vi "Fit ASCII Peak.vi"() -> ()   [LabVIEW 2016]
uses:
  <vilib>/Utility/file.llb/Read Delimited Spreadsheet (DBL).vi
  Smooth Background DBL.vi
  <vilib>/Analysis/NI_AALPro.lvlib
panel:
  in  "Use last fit as  guess":bool=TRUE
  in  "Function":enum16{"Gauss", "Lorentz"}(ring)
  out "errors":i32[](array[numeric])
  in  "Signal col":i32=2
  out "Fit":T1(array[cluster])
  in  "Repeat":i32
  in  "Guess":T1(array[cluster])
  in  "Window end":dbl=697.0
  in  "Window start":dbl=690.0
  in  "Filter background":bool=TRUE
  out "Result":T2
  out "error":i32
  out "XY Graph":cluster{"all rows":dbl[], "Data out":dbl[]}[](graph)
  in  "File Path Control":path
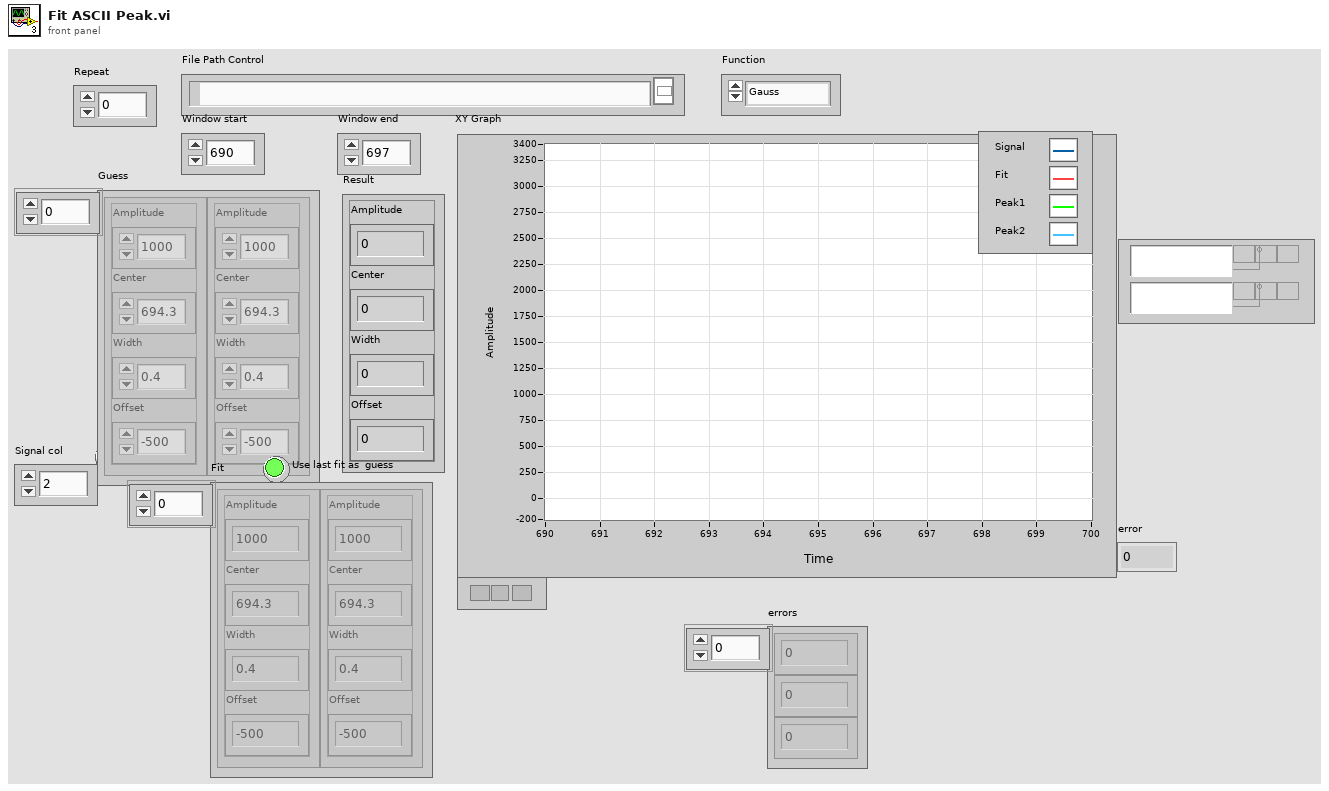
[diagram p1: front panel]
types:
  T1 = cluster{"Amplitude":dbl, "Center":dbl, "Width":dbl, "Offset":dbl}[]
  T2 = cluster{"Amplitude":dbl, "Center":dbl, "Width":dbl, "Offset":dbl}
  T3 = cluster{"amp min":dbl, "amp max":dbl, "center min":dbl, "center max":dbl, "deviation min":dbl, "deviation max":dbl, "offset min":dbl, "offset max":dbl}
  T4 = enum16{"Lowpass", "Highpass", "Bandpass", "Bandstop"}
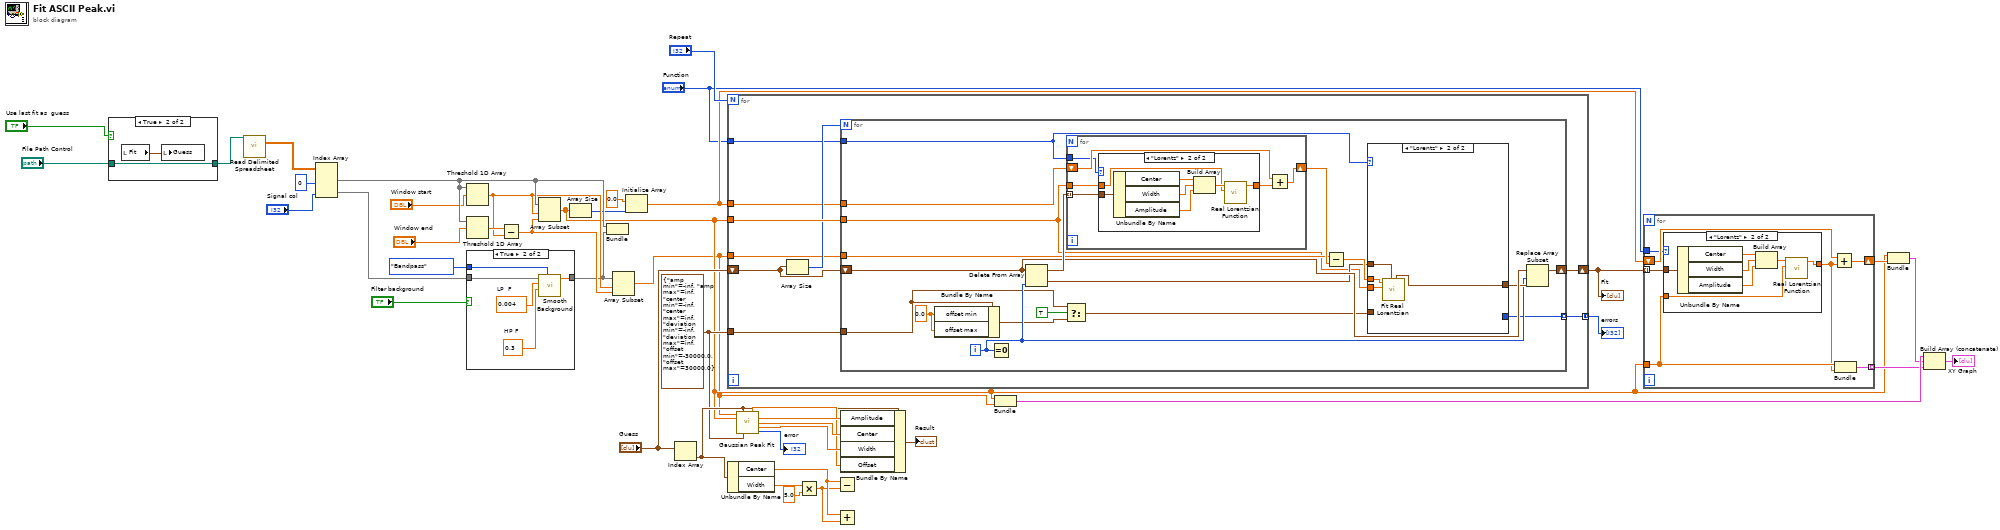
[diagram p0: block diagram]
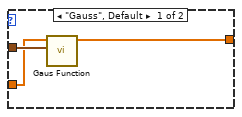
[diagram p3: hidden frame]
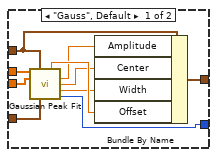
[diagram p4: hidden frame]
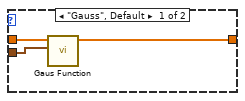
[diagram p5: hidden frame]
diagram:
  w13 = T3 {"amp min"=-inf, "amp max"=inf, "center min"=-inf, "center max"=inf, "deviation min"=-inf, "deviation max"=inf, "offset min"=-30000.0, "offset max"=30000.0} ("parameter bounds")
  n1 = case shown="True" "Use last fit as  guess" {
    tunnel: "File Path Control" -> [w44 w46]
    tunnel: [w44 w46] -> w1
    frame False {
    }
    frame True {
      n2 = local read "Fit"() -> (w45:T1)
      n3 = local write "Guess"(w45) -> ()
    }
  }
  n4 = call-poly <vilib>:"Read Delimited Spreadsheet.vi"("file path (dialog if empty)"=w1) -> ("all rows"=w43:dbl[][])  [unwired: 9 in, 5 out]
  n5 = Index Array(array=w43, index (col) #1=0 ("disabled index (col)"), index (col) #2="Signal col") -> (element #1=w35:dbl[], element #2=w37:dbl[])  [unwired: 2 in]
  n6 = Threshold 1D Array(2:"Window start", 3:w35) -> (0:w33:dbl)  [unwired: 1 in]
  n7 = Threshold 1D Array(2:"Window end", 3:w35) -> (0:w34:dbl)  [unwired: 1 in]
  n8 = case shown="True" "Filter background" {
    tunnel: T4."Bandpass" ("Type") -> [_ w52]
    tunnel: w37 -> [w47 w49]
    tunnel: [w47 w48] -> w31
    frame False {
    }
    frame True {
      w50 = 0.3  # HP F
      w51 = 0.004  # LP  F
      n9 = call-poly "Smooth Background.vi"("Type"=w52, "HP F"=w50, "LP  F"=w51, "Data"=w49) -> ("Data out"=w48:dbl[])  [unwired: 6 in, 1 out]
    }
  }
  n10 = Subtract(x=w34, y=w33) -> (x-y=w32:dbl)
  n11 = Array Subset(array=w35, index=w33, length=w32) -> (w8:dbl[])
  n12 = Array Size(array=w8) -> (size(s)=w16:i32)
  n13 = Bundle("all rows"=w35, "Data out"=w31) -> ()  [unwired: 1 in, 1 out]
  n14 = Array Subset(array=w31, index=w33, length=w32) -> (w6:dbl[])
  n15 = Initialize Array(0.0 ("element"), w16) -> (w10:dbl[])
  n16 = Index Array(array="Guess") -> (element=w18:T2)  [unwired: 1 in]
  n17 = for {
    N: "Repeat" -> [_]
    shift-right: [w56] -> w12
    shift-left: "Guess" -> [w60]
    tunnel: w8 -> [w61]
    tunnel: w10 -> [w58]
    tunnel: w6 -> [w57]
    tunnel: w13 -> [w55]
    tunnel: [w54] -> w5 mode=concatenating
    tunnel: "Function" -> [w53]
    n18 = Array Size(array=w60) -> (size(s)=w59:i32)
    n19 = for {
      N: w59 -> [_]
      tunnel: w61 -> [w63]
      tunnel: w58 -> [w78]
      tunnel: w57 -> [w76]
      shift-right: [w71] -> w56
      shift-left: w60 -> [w74]
      tunnel: w55 -> [w69]
      tunnel: [w65] -> w54 mode=indexing
      tunnel: w53 -> [w62]
      i -> [w70]
      w66 = 0.0
      n20 = Bundle By Name(cluster=w69, "offset min"=w66, "offset max"=w66) -> (w68:T3)
      n21 = Equal To 0?(x=w70) -> ()  [unwired: 1 out]
      n22 = Delete From Array(array=w74, index=w70) -> (deleted portion=w73:T2, array with subset deleted=w79:T1)  [unwired: 1 in]
      n23 = Select(t=w69, s=TRUE, f=w68) -> (s? t:f=w67:T3)
      n24 = for {
        tunnel: w79 -> [w99] mode=indexing
        tunnel: w63 -> [w98]
        shift-right: [w95] -> w77
        shift-left: w78 -> [w97]
        tunnel: w62 -> [w94]
        n25 = case shown="\"Lorentz\"" w94 {
          tunnel: w99 -> [w102 w106]
          tunnel: w98 -> [w101 w103]
          tunnel: [w100 w105] -> w96
          frame "Gauss", Default {
            n26 = call "Gaus Function.vi"("Fit params"=w102, "X"=w101) -> ("Y"=w100:dbl[])  [unwired: 9 in]
          }
          frame "Lorentz" {
            n27 = Unbundle By Name(w106) -> ("Center"=w109:dbl, "Width"=w108:dbl, "Amplitude"=w107:dbl)
            n28 = Build Array(w109, w108, w107) -> (w104:dbl[])
            n29 = call "Real Lorentzian Function.vi"("X"=w103, "a"=w104) -> ("f(X,a)"=w105:dbl[])  [unwired: 2 in, 2 out]
          }
        }
        n30 = Add(x=w97, y=w96) -> (x+y=w95:dbl[])
      }
      n31 = Subtract(x=w76, y=w77) -> (x-y=w75:dbl[])
      n32 = case shown="\"Lorentz\"" w62 {
        tunnel: w75 -> [w89 w93]
        tunnel: w73 -> [w88 w91]
        tunnel: [w83 w90] -> w72
        tunnel: w67 -> [w82 _]
        tunnel: [w81 _] -> w65
        tunnel: w63 -> [w80 w92]
        frame "Gauss", Default {
          n33 = call <vilib>:"Gaussian Peak Fit.vi"("Y"=w89, "initial guess"=w88, "X"=w80, "parameter bounds"=w82) -> ("offset"=w87:dbl, "amplitude"=w86:dbl, "center"=w85:dbl, "standard deviation"=w84:dbl, "error"=w81:i32)  [unwired: 5 in, 2 out]
          n34 = Bundle By Name(cluster=w88, "Amplitude"=w86, "Center"=w85, "Width"=w84, "Offset"=w87) -> (w83:T2)
        }
        frame "Lorentz" {
          n35 = call "Fit Real Lorentzian.vi"("Initial guess"=w91, "X"=w92, "Y"=w93) -> ("Fit"=w90:T2)  [unwired: 8 in]
        }
      }
      n36 = Replace Array Subset(array=w74, new element=w72, index=w70) -> (w71:T1)
    }
  }
  "Fit" <- w12
  "errors" <- w5
  n37 = Unbundle By Name(w18) -> ("Center"=w29:dbl, "Width"=w30:dbl)
  n38 = call <vilib>:"Gaussian Peak Fit.vi"("Y"=w6, "initial guess"=w18, "X"=w8, "parameter bounds"=w13) -> ("offset"=w23:dbl, "amplitude"=w26:dbl, "center"=w25:dbl, "standard deviation"=w24:dbl, "error"=→"error":i32)  [unwired: 5 in, 2 out]
  n39 = Multiply(x=w30, y=5.0) -> (x*y=w27:dbl)
  n40 = Subtract(x=w29, y=w27) -> ()  [unwired: 1 out]
  n41 = Add(x=w29, y=w27) -> ()  [unwired: 1 out]
  n42 = Bundle By Name(cluster=w18, "Amplitude"=w26, "Center"=w25, "Width"=w24, "Offset"=w23) -> (→"Result":T2)
  n43 = Bundle(w8, w6) -> (w38:cluster{dbl[], dbl[]})  [unwired: 1 in]
  n44 = for {
    tunnel: [w116] -> w11 mode=indexing
    tunnel: w8 -> [w113]
    tunnel: w12 -> [w111] mode=indexing
    shift-right: [w114] -> w9
    shift-left: w10 -> [w115]
    tunnel: "Function" -> [w110]
    n45 = case shown="\"Lorentz\"" w110 {
      tunnel: w111 -> [w119 w123]
      tunnel: w113 -> [w118 w121]
      tunnel: [w117 w122] -> w112
      frame "Gauss", Default {
        n46 = call "Gaus Function.vi"("Fit params"=w119, "X"=w118) -> ("Y"=w117:dbl[])  [unwired: 9 in]
      }
      frame "Lorentz" {
        n47 = Unbundle By Name(w123) -> ("Center"=w126:dbl, "Width"=w125:dbl, "Amplitude"=w124:dbl)
        n48 = Build Array(w126, w125, w124) -> (w120:dbl[])
        n49 = call "Real Lorentzian Function.vi"("X"=w121, "a"=w120) -> ("f(X,a)"=w122:dbl[])  [unwired: 2 in, 2 out]
      }
    }
    n50 = Add(x=w115, y=w112) -> (x+y=w114:dbl[])
    n51 = Bundle(w113, "f(X,a)"=w112) -> (w116:cluster{dbl[], "f(X,a)":dbl[]})  [unwired: 1 in]
  }
  n52 = Bundle(w8, w9) -> (w7:cluster{dbl[], dbl[]})  [unwired: 1 in]
  n53 = Build Array (concatenate)(w38, w7, w11) -> (→"XY Graph":cluster{dbl[], "f(X,a)":dbl[]}[])
